vi "Secure-Release Region.vi"(7 "Action":enum16{"Secure", "Release"}(ring), 8 "error in (no error)":errorcluster, 10 "Control In":T1={"I-O.lvclass"=refnum, "Motion.lvclass"=refnum, "Dispenser.lvclass"=refnum}, 11 "Carrier Tray in":refnum<class "Assembly Tray.lvclass">) -> (0 "error out":errorcluster, 2 "Control Out":T1, 3 "Carrier Tray out":refnum<class "Assembly Tray.lvclass">)   [LabVIEW 2016, in "Assembly Tray.lvclass"]
uses:
  Assembly Tray.lvclass
  D:/UCSB-Gantry/V5/Classes/Workspace/Fixture.lvclass
  Controller/Controllers.ctl
  Controller/I-O/I-O.lvclass
  Controller/Motion/A3200/A3200.lvclass
  Controller/Dispenser/Dispenser.lvclass
  Controller/Motion/Motion.lvclass
  Fixture.lvclass/Fixture.ctl
  Assembly Tray.lvclass/Assembly Tray.ctl
  Fixture.lvclass
  Controller/Controller.lvclass
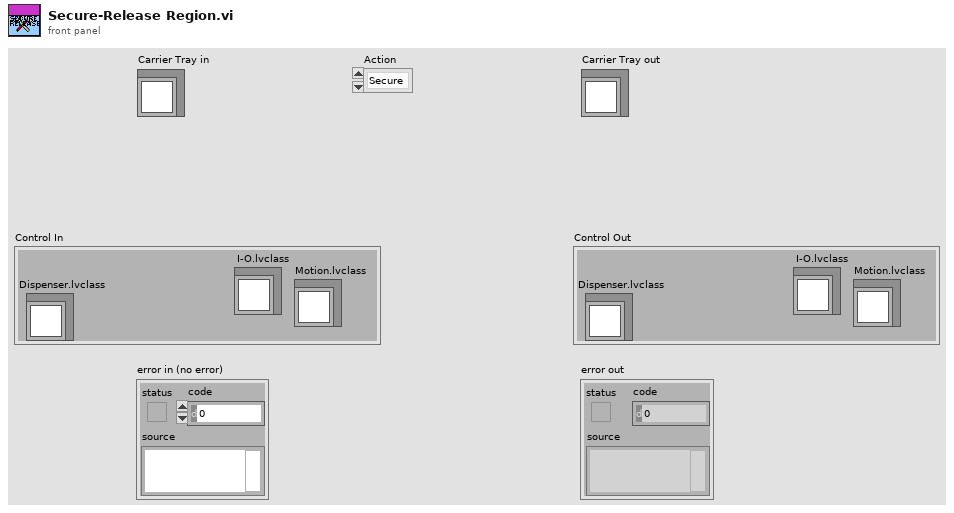
[diagram p1: front panel]
types:
  T1 = typedef "Controller.lvclass/Controllers.ctl" = cluster{"I-O.lvclass":refnum<class "I-O.lvclass">, "Motion.lvclass":refnum<class "Motion.lvclass">, "Dispenser.lvclass":refnum<class "Dispenser.lvclass">}
  T2 = typedef "I-O.lvclass/Pin Map.ctl" = cluster{"Region Valves":i32[], "Extra Valves":dbl[][][], "Tool Primary Valve":i32, "Tool Secondary Valve":i32, "Region Sensors":i32[], "Extra Sensors":dbl[][][], "Tool Primary Sensor":dbl, "Tool Secondary Sensor":dbl, "Compression Sensor":dbl, "5V":i32}
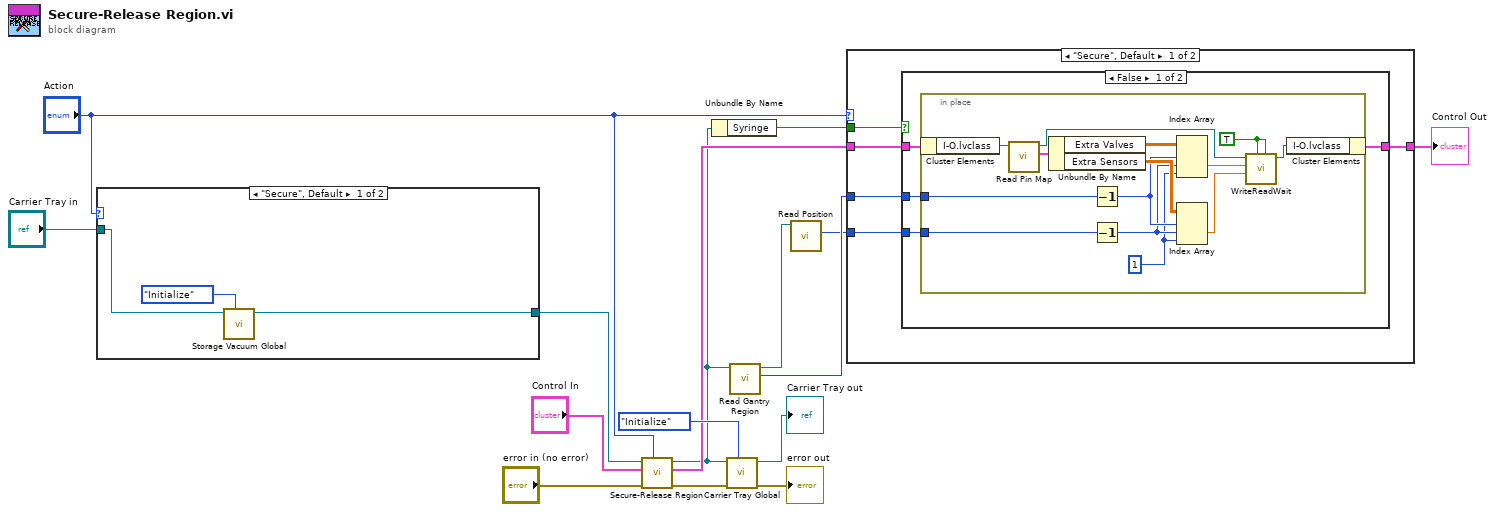
[diagram p0: block diagram]
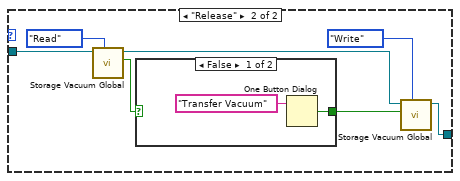
[diagram p4: hidden frame]
diagram:
  n1 = case shown="\"Secure\", Default" "Action" {
    tunnel: [w18 w21] -> w10
    tunnel: "Carrier Tray in" -> [w17 w20]
    frame "Secure", Default {
      n2 = call "Storage Vacuum Global.vi"("Action"=enum16{"Initialize", "Read", "Write"}."Initialize", "Carrier Tray.lvclass"=w17) -> ("Carrier Tray.lvclass 2"=w18:refnum<class "Assembly Tray.lvclass">)  [unwired: 7 in, 2 out]
    }
    frame "Release" {
      n3 = call "Storage Vacuum Global.vi"("Action"=enum16{"Initialize", "Read", "Write"}."Read", "Carrier Tray.lvclass"=w20) -> ("Read"=w26:bool, "Carrier Tray.lvclass 2"=w22:refnum<class "Assembly Tray.lvclass">)  [unwired: 7 in, 1 out]
      n4 = case shown="False" w26 {
        selector: w26 -> [_ w29]
        tunnel: [w27 w29] -> w23
        frame False {
          n5 = One Button Dialog(message="Transfer Vacuum") -> (true=w27:bool)  [unwired: 1 in]
        }
        frame True {
        }
      }
      n6 = call "Storage Vacuum Global.vi"("Action"=enum16{"Initialize", "Read", "Write"}."Write", "Write"=w23, "Carrier Tray.lvclass"=w22) -> ("Carrier Tray.lvclass 2"=w21:refnum<class "Assembly Tray.lvclass">)  [unwired: 6 in, 2 out]
    }
  }
  n7 = call-parent "Secure-Release Region.vi"("Action"="Action", "error in (no error)"="error in (no error)", "Control In"="Control In", "Fixture in"=w10) -> ("error out"=w14:errorcluster, "Control Out"=w7:T1, "Fixture out"=w6:refnum<class "Assembly Tray.lvclass">)  [unwired: 5 in]
  n8 = Unbundle By Name(w6) -> ("Syringe"=w8:bool)
  n9 = call "Carrier Tray Global.vi"("Action"=enum16{"Initialize", "Read", "Write"}."Initialize", "error in (no error)"=w14, "Carrier Tray.lvclass"=w6) -> ("error out"=→"error out":errorcluster, "Carrier Tray.lvclass 2"=→"Carrier Tray out":refnum<class "Assembly Tray.lvclass">)  [unwired: 6 in, 1 out]
  n10 = call "Read Gantry Region.vi"("Fixture in"=w6) -> ("Gantry Region"=w4:i32, "Fixture out"=w5:refnum<class "Assembly Tray.lvclass">)  [unwired: 8 in, 1 out]
  n11 = call "Read Position.vi"("Fixture in"=w5) -> ("Position"=w3:i32)  [unwired: 8 in, 2 out]
  n12 = case shown="\"Secure\", Default" "Action" {
    tunnel: w8 -> [w34 _]
    tunnel: w7 -> [w33 w54]
    tunnel: w4 -> [w32 _]
    tunnel: w3 -> [w31 _]
    tunnel: [w30 w54] -> w2
    frame "Secure", Default {
      n13 = case shown="False" w34 {
        tunnel: w33 -> [w38 w53]
        tunnel: w32 -> [w37 _]
        tunnel: w31 -> [w36 _]
        tunnel: [w35 w53] -> w30
        frame False {
          n14 = in-place {
            in-place-border: w37 -> [w45]
            in-place-border: w36 -> [w43]
            w41 = 1
            w47 = TRUE
            n15 = in-place-cluster #1(w38) -> ("I-O.lvclass"=w52:refnum<class "I-O.lvclass">)
            n16 = call-dynamic "Read Pin Map.vi"("I-O in"=w52) -> ("Pin Map 2"=w51:T2, "I-O out"=w48:refnum<class "I-O.lvclass">)  [unwired: 8 in, 1 out]
            n17 = Unbundle By Name(w51) -> ("Extra Valves"=w50:dbl[][][], "Extra Sensors"=w49:dbl[][][])
            n18 = Decrement(x=w45) -> (x-1=w44:i32)
            n19 = Decrement(x=w43) -> (x-1=w42:i32)
            n20 = Index Array(array=w50, index (dim 0)=w44, index (dim 1)=w42, index (dim 2)=w41) -> (element=w40:dbl)
            n21 = Index Array(array=w49, index (dim 0)=w44, index (dim 1)=w42, index (dim 2)=w41) -> (element=w39:dbl)
            n22 = call "WriteReadWait.vi"("Read Value"=w47, "Write Value"=w47, "Read"=w39, "Write"=w40, "I-O in"=w48) -> ("I-O out"=w46:refnum<class "I-O.lvclass">)  [unwired: 5 in, 1 out]
            n23 = in-place-cluster #1("I-O.lvclass"=w46) -> (w35:T1)
          }
        }
        frame True {
        }
      }
    }
    frame "Release" {
    }
  }
  "Control Out" <- w2
